vi "TipStrip Daemon.vi"(11 "TipStripOOPanel.lvlib:TipPanelHandle.lvclass":refnum<class "TipPanelHandle.lvclass">) -> ()   [LabVIEW 2021, in "TipStripOOPanel.lvlib" / "TipPanelHandle.lvclass"]
uses:
  TipPanelHandle.lvclass
  SubVIs/refs.ctl
  TipPanelHandle.lvclass/TipPanelHandle.ctl
  <vilib>/Utility/inputDevices.llb/closeMouse.vi
  <vilib>/Futures/Futures/Promise/Promise.lvclass
  TipStripOOPanel.lvlib
  <vilib>/IlluminatedG/IG OOPanel/OOPanel/Manager/Manager.lvclass
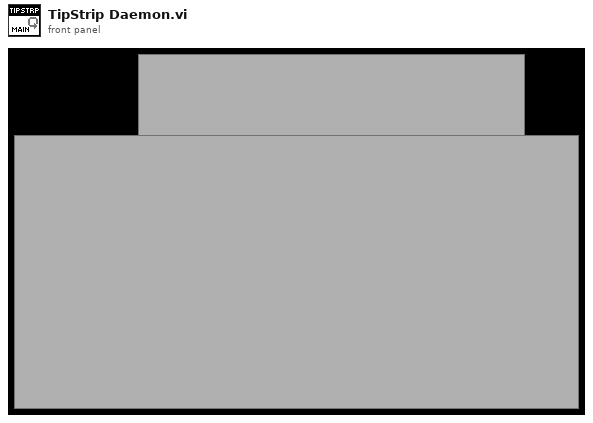
[diagram p1: front panel]
types:
  T1 = typedef "TipStripOOPanel.lvlib/refs.ctl" = cluster{"Front Panel":refnum<vi>, "VI":refnum<vi>, "Sub Panel":refnum<vi>}
  T2 = typedef "TipStripOOPanel.lvlib/tipstrip_screens.ctl" = cluster{"X0":i32, "Y0":i32, "X1":i32, "Y1":i32}
  T3 = typedef "TipStripOOPanel.lvlib/Loop Data Parent.ctl" = cluster{"PanelMap":T4, "PanelMgr":refnum<class "Manager.lvclass">, "ActiveTipPanel":refnum<class "TipPanel.lvclass">, "visible?":bool, "Refs":T1, "Bounds":T6, "content":T7}
  T4 = typedef "TipStripOOPanel.lvlib/PanelMap.ctl" = map{refnum<class "TipPanel.lvclass">, T5}
  T5 = typedef "TipStripOOPanel.lvlib/PanelMapData.ctl" = cluster{"Mgr.Panel":refnum<class "TipPanel.lvclass">, "ToPanel:New":refnum<user-event>}
  T6 = typedef "LVRectTypeDef.ctl" = cluster{"Left":i16, "Top":i16, "Right":i16, "Bottom":i16}
  T7 = typedef "LVBoundsTypeDef.ctl" = cluster{"Width":u32, "Height":u32}
  T8 = typedef "TipStripOOPanel.lvlib/tipstrip action.ctl" = enum16{"hide", "show"}
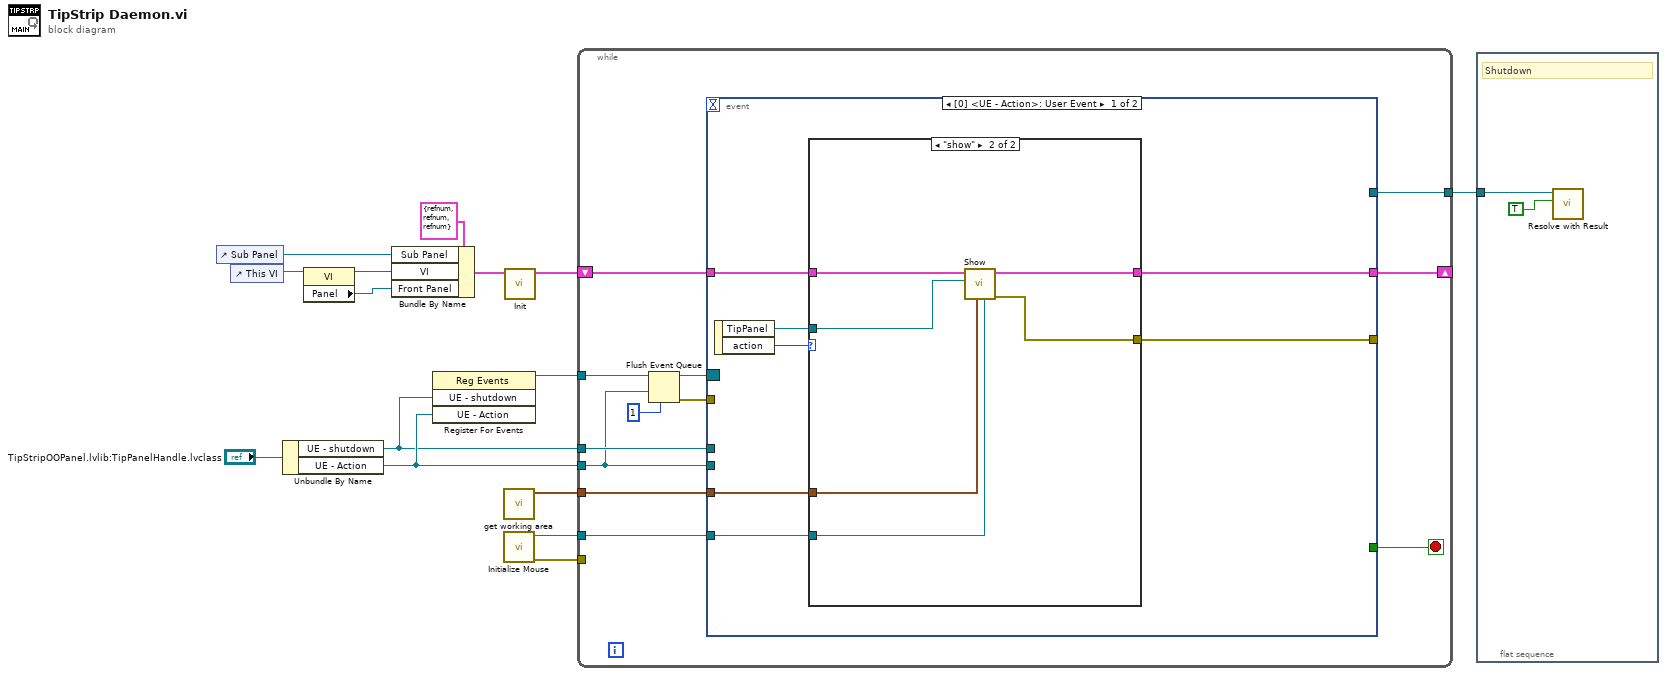
[diagram p0: block diagram]
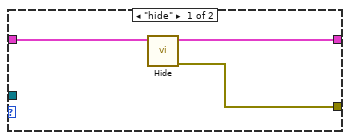
[diagram p2: hidden frame]
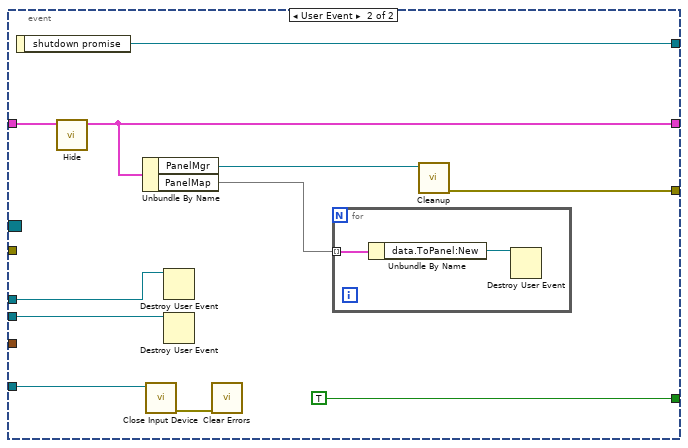
[diagram p3: hidden frame]
diagram:
  n1 = control-ref of="Sub Panel"() -> (w7:refnum<vi>)
  n2 = control-ref of="This VI"() -> (w12:refnum<vi>)
  n3 = Unbundle By Name("TipStripOOPanel.lvlib:TipPanelHandle.lvclass") -> ("UE - shutdown"=w1:refnum<user-event>, "UE - Action"=w3:refnum<user-event>)
  n4 = property class="VI"(reference=w12) -> (reference out=w8:refnum<vi>, "Panel"=w10:refnum<vi>)  [unwired: 1 in, 1 out]
  n5 = Bundle By Name(cluster=T1 {"Front Panel"=refnum, "VI"=refnum, "Sub Panel"=refnum} ("Cluster"), "Sub Panel"=w7, "VI"=w8, "Front Panel"=w10) -> (w6:T1)
  n6 = register-events(w1, w3) -> (reference out=w15:refnum<event-registration>)  [unwired: 2 in, 1 out]
  n7 = call "get working area.vi"() -> ("screens"=w9:T2[])  [unwired: 10 in, 1 out]
  n8 = call <vilib>:"Initialize Mouse.vi"() -> ("error out"=w13:errorcluster, "device ID"=w14:refnum<k1>)  [unwired: 10 in]
  n9 = call "Init.vi"("Refs"=w6) -> ("Loop data init"=w5:T3)  [unwired: 10 in]
  n10 = while {
    tunnel: w15 -> [w22]
    tunnel: w14 -> [w27]
    tunnel: w13 -> [_]
    shift-right: [w25] -> _
    shift-left: w5 -> [w26]
    tunnel: w9 -> [w24]
    tunnel: w3 -> [w16]
    tunnel: [w18] -> w2
    tunnel: w1 -> [w17]
    stop <- w23 stop-if-true
    n11 = Flush Event Queue(0:w22, 2:w16, 5:1 ("keep most recent")) -> (8:w21:refnum<event-registration>, 11:w19:errorcluster)  [unwired: 3 in, 1 out]
    n12 = event shown="[0] <UE - Action>: User Event" {
      selector: w21 -> [_ _]
      dyn-events: _ -> [_ _]
      timeout: _ -> [_ _]
      tunnel: w27 -> [w33 w53]
      tunnel: w26 -> [w32 w52]
      tunnel: [w31 w50] -> w25
      tunnel: w24 -> [w30 _]
      tunnel: [_ TRUE] -> w23
      tunnel: [w28 w47] -> _
      tunnel: w19 -> [_ _]
      tunnel: [_ w46] -> w18
      tunnel: w17 -> [_ w45]
      tunnel: w16 -> [_ w44]
      event User Event {
        n13 = event-data() -> ("TipPanel"=w29:refnum<class "TipPanel.lvclass">, "action"=w34:T8)  [unwired: 1 in]
        n14 = case shown="\"show\"" w34 {
          tunnel: w33 -> [_ w41]
          tunnel: w32 -> [w37 w43]
          tunnel: [w36 w40] -> w31
          tunnel: w30 -> [_ w42]
          tunnel: w29 -> [_ w38]
          tunnel: [w35 w39] -> w28
          frame "hide" {
            n15 = call "Hide.vi"("loop data in"=w37) -> ("error out"=w35:errorcluster, "loop data out"=w36:T3)  [unwired: 9 in]
          }
          frame "show" {
            n16 = call "Show.vi"("device ID"=w41, "screens"=w42, "TipPanel"=w38, "loop data in"=w43) -> ("error out"=w39:errorcluster, "loop data out"=w40:T3)  [unwired: 6 in]
          }
        }
      }
      event User Event {
        n17 = event-data() -> ("shutdown promise"=w46:refnum<class "Promise.lvclass">)  [unwired: 1 in]
        n18 = call "Hide.vi"("loop data in"=w52) -> ("loop data out"=w50:T3)  [unwired: 9 in, 1 out]
        n19 = Unbundle By Name(w50) -> ("PanelMgr"=w48:refnum<class "Manager.lvclass">, "PanelMap"=w49:T4)
        n20 = call-poly <vilib>:"Close Input Device.vi"("device ID"=w53) -> ("error out"=w54:errorcluster)  [unwired: 9 in]
        n21 = Destroy User Event(user event=w45) -> ()  [unwired: 1 in, 1 out]
        n22 = Destroy User Event(user event=w44) -> ()  [unwired: 1 in, 1 out]
        n23 = call <vilib>:"Clear Errors.vi"("error in (no error)"=w54) -> ()  [unwired: 5 in, 2 out]
        n24 = for {
          tunnel: w49 -> [w56] mode=indexing
          n25 = Unbundle By Name(w56) -> ("data.ToPanel:New"=w55:refnum<user-event>)
          n26 = Destroy User Event(user event=w55) -> ()  [unwired: 1 in, 1 out]
        }
        n27 = call <vilib>:"Cleanup.vi"("Manager in"=w48) -> ("error out"=w47:errorcluster)  [unwired: 8 in, 2 out]
      }
    }
  }
  n28 = flat-sequence {
    tunnel: w2 -> [w58]
    frame #0 {
      # "Shutdown"
      n29 = call <vilib>:"Resolve with Result.vi"("Result"=TRUE, "Promise in"=w58) -> ()  [unwired: 9 in, 1 out]
    }
  }
